vi "Move.vi"(6 "Mode":enum16{"Relative", "Absolute"}(ring), 7 "Correlation ID":u32, 8 "error in (no error)":errorcluster, 9 "Value (mm)":dbl format="%#_13g", 10 "Axis":T1=enum."Y", 11 "Stage Controller in":refnum<class "Stage Controller.lvclass">) -> (0 "error out":errorcluster, 3 "Stage Controller out":refnum<class "Stage Controller.lvclass">)   [LabVIEW 2023, in "Stage Controller.lvlib" / "Stage Controller.lvclass"]
uses:
  Stage Controller.lvclass
  Stage Controller.lvclass/Stage Controller.ctl
  Application Messages/Automation_TaskCompleted Msg/Automation_TaskCompleted Msg.lvclass
  <vilib>/ActorFramework/Actor/Actor.lvclass
  C:/Program Files/National Instruments/LabVIEW 2023/vi.lib/ActorFramework/Actor/Actor.lvclass
  Stage Axis.ctl
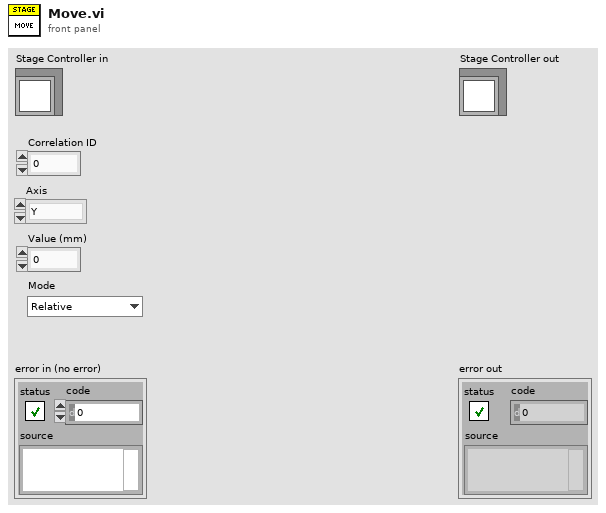
[diagram p1: front panel]
types:
  T1 = typedef "Stage Controller.lvlib/Stage Controller.lvclass/Stage Axis.ctl" = enum16{"unspecified", "X", "Y", "Z"}
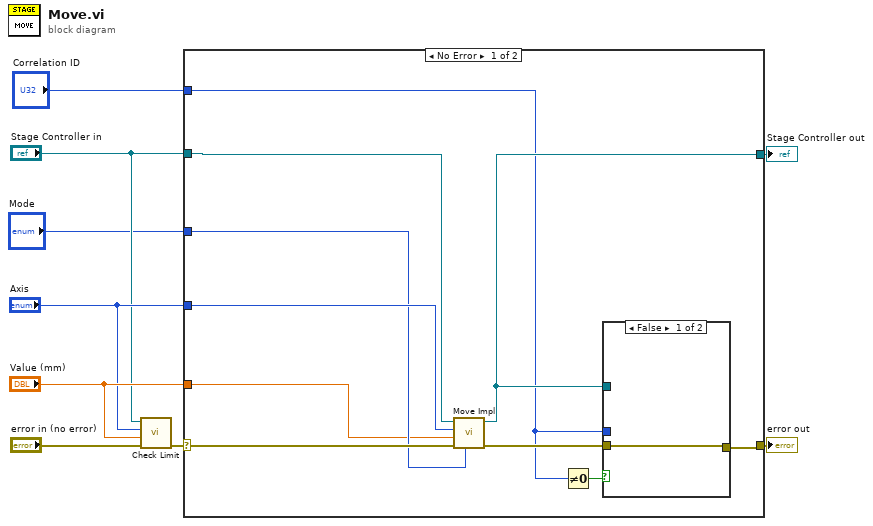
[diagram p0: block diagram]
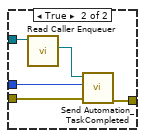
[diagram p2: hidden frame]
diagram:
  n1 = call-dynamic "Check Limit.vi"("error in (no error)"="error in (no error)", "Distance (mm)"="Value (mm)", "Axis"="Axis", "Stage Controller in"="Stage Controller in") -> ("error out"=w7:errorcluster)  [unwired: 6 in, 1 out]
  n2 = case shown="No Error" w7 {
    selector: w7 -> [w19 w27]
    tunnel: [w13 w27] -> w9
    tunnel: [w12 w26] -> w8
    tunnel: "Stage Controller in" -> [w18 w26]
    tunnel: "Value (mm)" -> [w15 _]
    tunnel: "Axis" -> [w17 _]
    tunnel: "Mode" -> [w16 _]
    tunnel: "Correlation ID" -> [w10 _]
    frame No Error {
      n3 = call-dynamic "Move Impl.vi"("Mode"=w16, "error in (no error)"=w19, "Value (mm)"=w15, "Axis"=w17, "Stage Controller in"=w18) -> ("error out"=w14:errorcluster, "Stage Controller out"=w12:refnum<class "Stage Controller.lvclass">)  [unwired: 5 in]
      n4 = Not Equal To 0?(x=w10) -> (x != 0?=w11:bool)
      n5 = case shown="False" w11 {
        tunnel: w14 -> [w20 w25]
        tunnel: [w20 w24] -> w13
        tunnel: w12 -> [_ w23]
        tunnel: w10 -> [_ w21]
        frame False {
        }
        frame True {
          n6 = call <vilib>:"Read Caller Enqueuer.vi"("Actor"=w23) -> ("Caller Enqueuer"=w22:refnum<class "Message Enqueuer.lvclass">)  [unwired: 10 in]
          n7 = call "Send Automation_TaskCompleted.vi"("error in (no error)"=w25, "Correlation ID"=w21, "Message Enqueuer"=w22) -> ("error out"=w24:errorcluster)  [unwired: 7 in, 1 out]
        }
      }
    }
    frame Error {
    }
  }
  "error out" <- w9
  "Stage Controller out" <- w8
